vi "MicroStruct-XY.vi"() -> ()   [LabVIEW 2014]
doc: "Newport Motion Controler\nThis program make lines structure\n\nAndré Romero - 2020\nandretec@ifsc.usp.br"
uses:
  <vilib>/Platform/TimedLoop/XDataNode/timing_clust.ctl
  <vilib>/Platform/TimedLoop/XDataNode/nitl_modes.ctl
  <vilib>/Platform/TimedLoop/XDataNode/wakeup.ctl
  Basic-VIs/Global Motor Axis.vi
  <vilib>/Platform/TimedLoop/XDataNode/XDataNode.xnode
  <userlib>/Newport ESP301/Newport ESP301.lvlib
  <vilib>/Platform/TimedLoop/XDataNode/XDNodeRunTimeDep.lvlib
panel:
  out "Abort":bool
  out "current cycle":i32=1
  in  "Swap motor":bool=TRUE
  out "XY Graph":cluster{dbl[], dbl[]}(graph)={[0.0, 0.0, 0.002, 0.0105, 0.0215, 0.037, 0.0555, 0.075, 0.096, 0.116, 0.136, 0.156, 0.176, 0.1955, 0.216, 0.236, 0.256, 0.276, 0.2965, 0.3165, 0.336, 0.3565, 0.3755, 0.3965, 0.4165, 0.4365, 0.4565, 0.477, 0.4965, 0.5165, 0.5365, 0.557, 0.5765, 0.597, 0.617, 0.6365, 0.6565, 0.6765, 0.697, 0.717, 0.737, 0.757, 0.777, 0.797, 0.8165, 0.8375, 0.8575, 0.877, 0.897, 0.9175, 0.937, 0.9575, 0.977, 0.9975, 1.0005, 1.0005, 1.0, 0.997, 0.9885, 0.9775, 0.9615, 0.9435, 0.923, 0.903, 0.883, 0.863, 0.843, 0.823, 0.8035, 0.783, 0.763, 0.743, 0.723, 0.7035, 0.683, 0.6635, 0.643, 0.6235, 0.603, 0.583, 0.563, 0.543, 0.523, 0.5025, 0.483, 0.463, 0.443, 0.4225, 0.403, 0.3825, 0.363, 0.3425, 0.323, 0.303, 0.2825, 0.2625, 0.2425, 0.2225, 0.202, 0.183, 0.162, 0.1425, 0.1225, 0.1025, 0.082, 0.0625, 0.042, 0.0225, 0.002, -0.0005, -0.0005, 0.0, 0.0035, 0.013, 0.025, 0.0415, 0.06, 0.08, 0.1005, 0.1205, 0.1405, 0.1605, 0.18, 0.2005, 0.2205, 0.2405, 0.2605, 0.28, 0.3, 0.3205, 0.3405, 0.3605, 0.3805, 0.4005, 0.4205, 0.4405, 0.4605, 0.4805, 0.5005, 0.52, 0.541, 0.5605, 0.58, 0.6005, 0.6205, 0.6405, 0.6605, 0.6805, 0.7005, 0.7205, 0.7405, 0.7605, 0.7805, 0.8005, 0.8205, 0.8405, 0.8605, 0.8805, 0.9005, 0.92, 0.94, 0.96, 0.9805, 1.0005, 1.0005, 1.0005, 0.9995, 0.993, 0.984, 0.9705, 0.9535, 0.9335, 0.9135, 0.8935, 0.8735, 0.8535, 0.8335, 0.8135, 0.7935, 0.7735, 0.753, 0.7335, 0.713, 0.6935, 0.6735, 0.6535, 0.633, 0.6135], [0.0035, 0.0035, 0.0035, 0.0035, 0.0035, 0.0035, 0.0035, 0.0035, 0.0035, 0.0035, 0.0035, 0.0035, 0.0035, 0.0035, 0.0035, 0.0035, 0.0035, 0.0035, 0.0035, 0.0035, 0.0035, 0.0035, 0.0035, 0.0035, 0.0035, 0.0035, 0.0035, 0.0035, 0.0035, 0.0035, 0.0035, 0.0035, 0.0035, 0.0035, 0.0035, 0.0035, 0.0035, 0.0035, 0.0035, 0.0035, 0.0035, 0.0035, 0.0035, 0.0035, 0.0035, 0.0035, 0.0035, 0.0035, 0.0035, 0.0035, 0.0035, 0.0035, 0.0035, 0.0035, 0.0035, 0.004, 0.005, 0.0055, 0.0055, 0.0055, 0.0055, 0.006, 0.0055, 0.0055, 0.0055, 0.0055, 0.0055, 0.0055, 0.0055, 0.0055, 0.0055, 0.0055, 0.0055, 0.0055, 0.0055, 0.0055, 0.0055, 0.0055, 0.0055, 0.0055, 0.0055, 0.0055, 0.0055, 0.0055, 0.0055, 0.0055, 0.0055, 0.0055, 0.0055, 0.0055, 0.0055, 0.0055, 0.0055, 0.0055, 0.0055, 0.0055, 0.0055, 0.0055, 0.0055, 0.0055, 0.0055, 0.0055, 0.0055, 0.0055, 0.0055, 0.0055, 0.0055, 0.0055, 0.0055, 0.0055, 0.006, 0.0085, 0.0085, 0.0085, 0.0075, 0.0075, 0.0075, 0.007, 0.007, 0.0075, 0.0075, 0.0075, 0.0075, 0.0075, 0.0075, 0.0075, 0.0075, 0.0075, 0.0075, 0.0075, 0.0075, 0.0075, 0.0075, 0.0075, 0.0075, 0.0075, 0.0075, 0.0075, 0.0075, 0.0075, 0.0075, 0.0075, 0.0075, 0.0075, 0.0075, 0.0075, 0.0075, 0.0075, 0.0075, 0.0075, 0.0075, 0.0075, 0.0075, 0.0075, 0.0075, 0.0075, 0.0075, 0.0075, 0.0075, 0.0075, 0.0075, 0.0075, 0.0075, 0.0075, 0.0075, 0.0085, 0.01, 0.01, 0.01, 0.01, 0.01, 0.0095, 0.0095, 0.0095, 0.0095, 0.0095, 0.0095, 0.0095, 0.0095, 0.0095, 0.0095, 0.0095, 0.009, 0.009, 0.0095, 0.0095, 0.0095, 0.0095]}
  in  "N Cycles":i32=100 min=1
  in  "Acceleration (0 units/s²)":dbl=0.1 min=0.0 format="%#.4g"
  in  "Velocity (units/s)":dbl=0.1 min=0.0 format="%#.4g"
  in  "d (mm)":dbl=2.0
  in  "L (mm)":dbl=1.0
  out "X Position (mm)":dbl=0.6135 format="%.6g"
  out "Y Position (mm)":dbl=0.0095 format="%.6g"
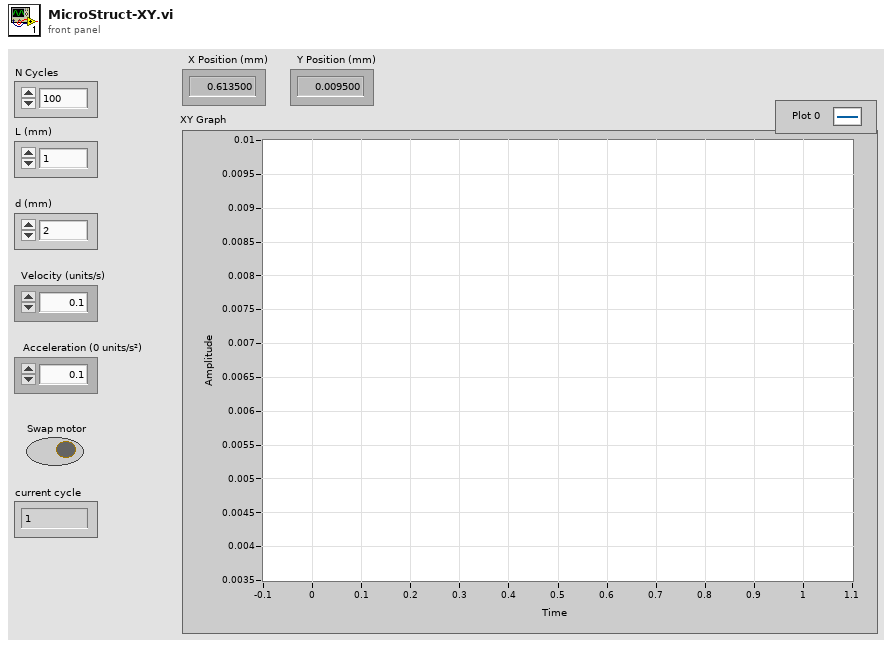
[diagram p1: front panel]
types:
  T1 = typedef "XDNodeRunTimeDep.lvlib/timing_clust.ctl" = cluster{"Expected End [f-1]":u64, "Actual End [f-1]":u64, "Finished Late? [f-1]":bool, "Expected End [i-1]":u64, "Actual End [i-1]":u64, "Finished Late? [i-1]":bool, "Expected Start [i]":u64, "Actual Start [i]":u64, "Expected Start [f]":u64, "Actual Start [f]":u64, "Source Name":string, "Structure Name":string, "Period":i64, "Deadline":i64, "Offset":i64, "Start":i64, "Priority":i32, "Timeout":i32, "Mode":T2, "Wakeup Reason":T3, "Error":errorcluster, "Source Type":string, "Secondary Source Type":string, "Global End Time":u64, "Global Start Time":u64, "Frame Duration":u64, "Iteration Duration":u64, "Assigned CPU":i32, "I/O Scan Engine Mode":u32}
  T2 = typedef "XDNodeRunTimeDep.lvlib/nitl_modes.ctl" = enum32{"No Change", "Process missed periods, maintain original phase", "Discard missed periods, maintain original phase", "Process missed periods, ignore original phase", "Discard missed periods, ignore original phase"}
  T3 = typedef "XDNodeRunTimeDep.lvlib/wakeup.ctl" = enum32{"Normal", "Aborted", "Asynchronous wakeup", "Timing source error", "Timed loop error", "Timeout"}
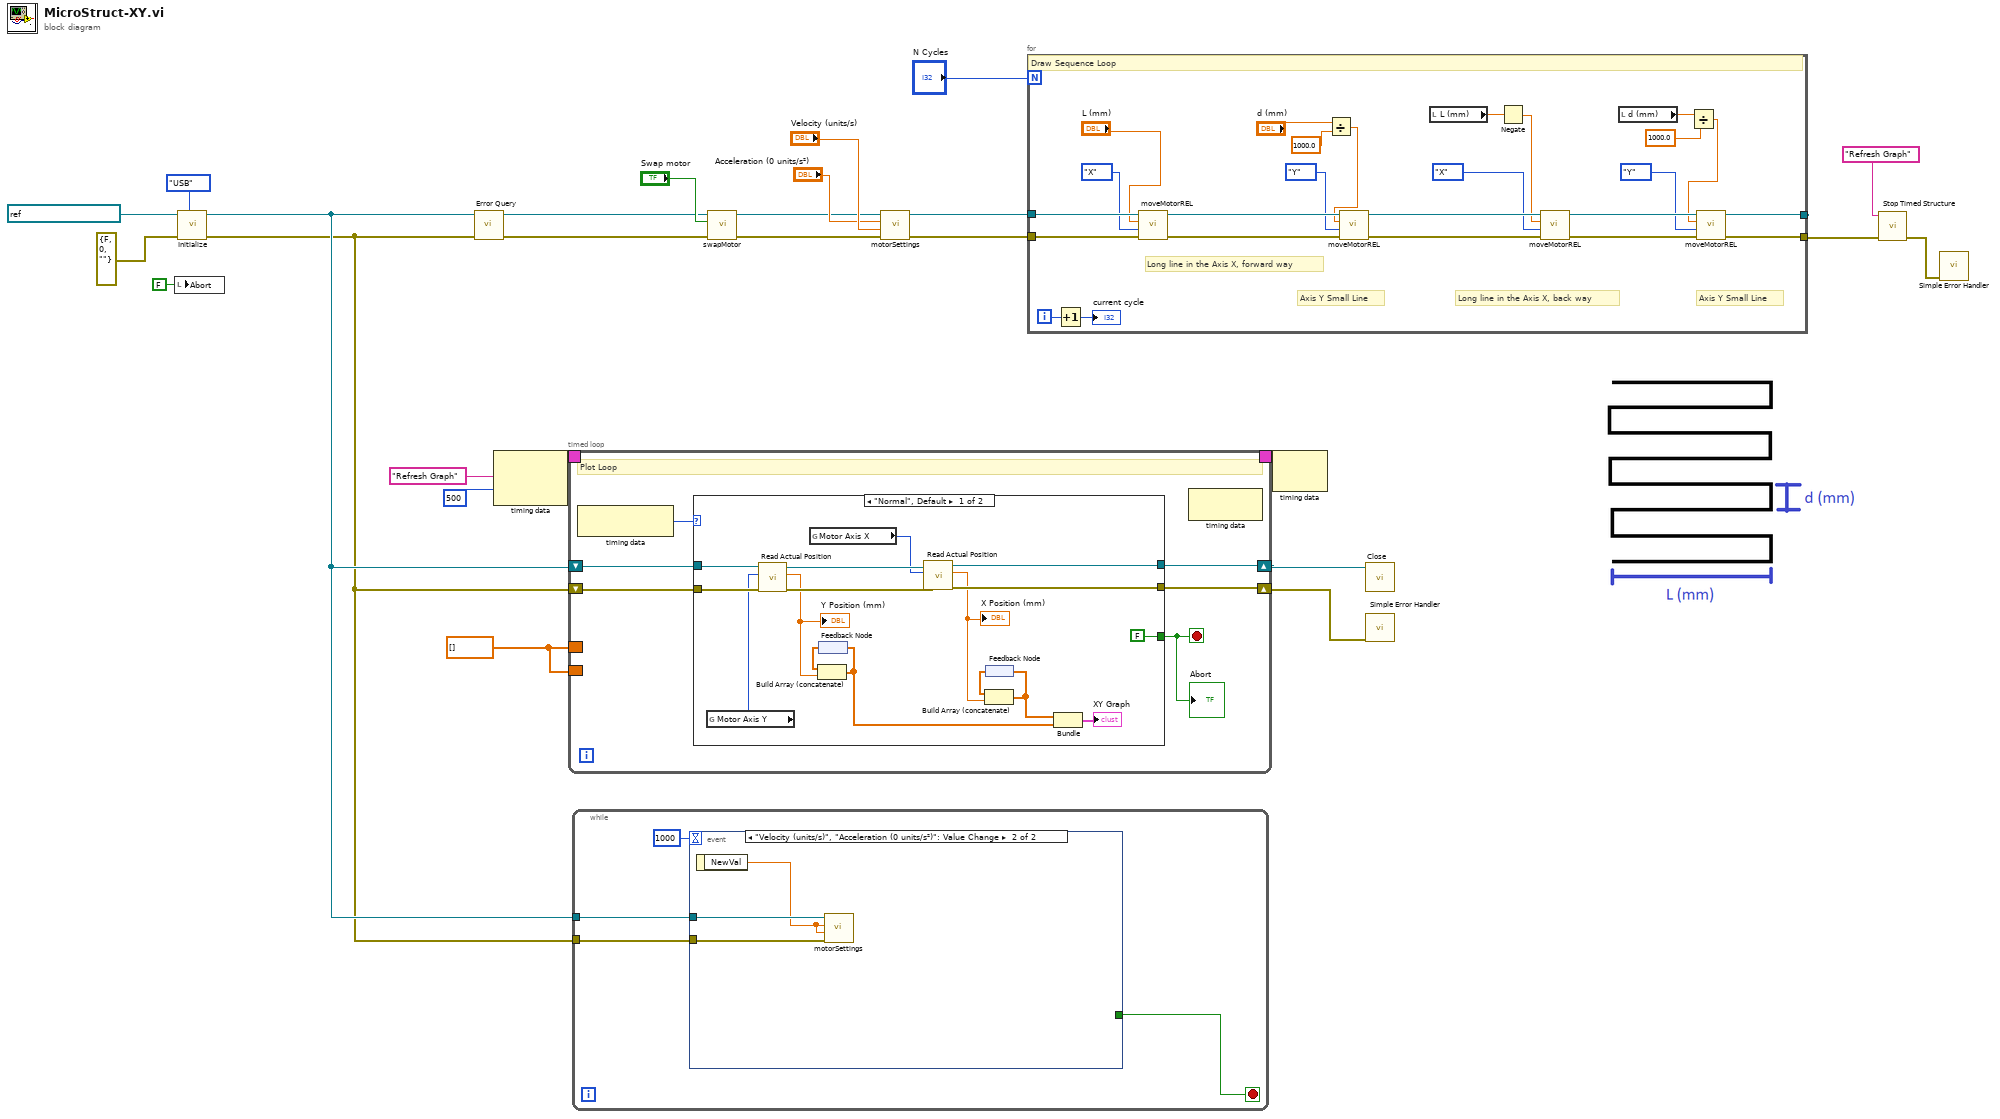
[diagram p0: block diagram]
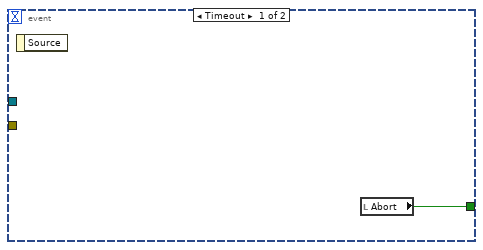
[diagram p2: hidden frame]
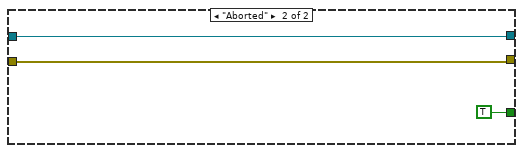
[diagram p3: hidden frame]
diagram:
  w14 = dbl[] []
  n1 = local write "Abort"(FALSE ("Abort")) -> ()
  n2 = call <userlib>:"Initialize.vi"("VISA resource name"=refnum<visa-resource-name> "ASRL3::INSTR" ("VISA resource name (duplicate)"), "error in (no error)"=errorcluster {"status"=FALSE, "code"=0, "source"=""}, "Serial Link (RS232)"=enum16{"RS232", "USB"}."USB") -> ("VISA resource name out"=w3:refnum<visa-resource-name>, "error out"=w2:errorcluster)  [unwired: 6 in]
  n3 = call <userlib>:"Error Query.vi"("error in (no error)"=w2, "VISA resource name"=w3) -> ("error out"=w9:errorcluster, "VISA resource name out"=w10:refnum<visa-resource-name>)  [unwired: 2 in, 2 out]
  n4 = node-c288("Refresh Graph" ("Structure Name"), i64 500 ("Period")) -> (w24:T1)
  n5 = timed-loop {
    timing: w24 -> [_]
    timing-out: [_] -> w23
    shift-right: [w30] -> w26
    shift-left: w3 -> [w32]
    shift-right: [w29] -> w25
    shift-left: w2 -> [w31]
    border: w14 -> [_]
    border: w14 -> [_]
    stop <- w27 stop-if-true
    # "Plot Loop"
    n6 = node-c288() -> (w28:T3)  [unwired: 1 in]
    n7 = case shown="\"Normal\", Default" w28 {
      tunnel: w32 -> [w48 w50]
      tunnel: w31 -> [w47 w49]
      tunnel: [w44 w50] -> w30
      tunnel: [w43 w49] -> w29
      tunnel: [FALSE TRUE] -> w27
      frame "Normal", Default {
        n8 = global read "Global Motor Axis.vi" "Motor Axis Y"() -> (w33:i32)
        n9 = call <userlib>:"Read Actual Position.vi"("error in (no error)"=w47, "Axis (1)"=w33, "VISA resource name"=w48) -> ("error out"=w45:errorcluster, "Position (units)"=w38:dbl, "VISA resource name out"=w46:refnum<visa-resource-name>)  [unwired: 2 in]
        "Y Position (mm)" <- w38
        n10 = global read "Global Motor Axis.vi" "Motor Axis X"() -> (w34:i32)
        n11 = feedback #1() -> (w41:dbl[])
        n12 = Build Array (concatenate)(w41, w38) -> (w36:dbl[])
        n13 = feedback-in #1(w36) -> ()
        n14 = call <userlib>:"Read Actual Position.vi"("error in (no error)"=w45, "Axis (1)"=w34, "VISA resource name"=w46) -> ("error out"=w43:errorcluster, "Position (units)"=w39:dbl, "VISA resource name out"=w44:refnum<visa-resource-name>)  [unwired: 2 in]
        "X Position (mm)" <- w39
        n15 = feedback #2() -> (w40:dbl[])
        n16 = Build Array (concatenate)(w40, w39) -> (w37:dbl[])
        n17 = feedback-in #2(w37) -> ()
        n18 = Bundle(w37, w36) -> (→"XY Graph":cluster{dbl[], dbl[]})  [unwired: 1 in]
      }
      frame "Aborted" {
      }
    }
    "Abort" <- w27
    n19 = node-c288() -> ()  [unwired: 1 in, 1 out]
  }
  n20 = while {
    tunnel: w3 -> [w58]
    tunnel: w2 -> [w57]
    stop <- w56 stop-if-true
    n21 = event shown="[1] \"Velocity (units/s)\", \"Acceleration (0 units/s²)\": Value Change" {
      selector: _ -> [_ _]
      dyn-events: _ -> [_ _]
      timeout: 1000 -> [_ _]
      tunnel: w58 -> [_ w61]
      tunnel: w57 -> [_ w62]
      tunnel: [w59 _] -> w56
      event Timeout {
        n22 = event-data() -> ()  [unwired: 1 in, 1 out]
        n23 = local read "Abort"() -> (w59:bool)
      }
      event "Velocity (units/s)", "Acceleration (0 units/s²)": Value Change {
        n24 = event-data() -> ("NewVal"=w60:dbl)  [unwired: 1 in]
        n25 = call "motorSettings.vi"("error in (no error)"=w62, "Velocity (units/s)"=w60, "Acceleration (0 units/s²)"=w60, "VISA Refnum in"=w61) -> ()  [unwired: 6 in, 2 out]
      }
    }
  }
  n26 = call "swapMotor.vi"("error in (no error)"=w9, "Swap motor"="Swap motor", "VISA Refnum in"=w10) -> ("error out"=w7:errorcluster, "VISA Refnum out"=w8:refnum<visa-resource-name>)  [unwired: 7 in]
  n27 = call "motorSettings.vi"("error in (no error)"=w7, "Velocity (units/s)"="Velocity (units/s)", "Acceleration (0 units/s²)"="Acceleration (0 units/s²)", "VISA Refnum in"=w8) -> ("error out"=w18:errorcluster, "VISA Refnum out"=w19:refnum<visa-resource-name>)  [unwired: 6 in]
  n28 = for {
    N: "N Cycles" -> [_]
    tunnel: w19 -> [w87]
    tunnel: w18 -> [w86]
    tunnel: [w75] -> _
    tunnel: [w74] -> w13
    i -> [w64]
    # "Axis Y Small Line"
    # "Long line in the Axis X, back way"
    # "Axis Y Small Line"
    # "Long line in the Axis X, forward way"
    # "Draw Sequence Loop"
    n29 = Increment(x=w64) -> (x+1=→"current cycle":i32)
    n30 = call "moveMotorREL.vi"("error in (no error)"=w86, "Axis"=enum16{"X", "Y"}."X", "L (mm)"="L (mm)", "VISA Refnum in"=w87) -> ("error out"=w83:errorcluster, "VISA Refnum out"=w84:refnum<visa-resource-name>)  [unwired: 6 in]
    n31 = Divide(x="d (mm)", y=1000.0 ("x")) -> (x/y=w68:dbl)
    n32 = call "moveMotorREL.vi"("error in (no error)"=w83, "Axis"=enum16{"X", "Y"}."Y", "L (mm)"=w68, "VISA Refnum in"=w84) -> ("error out"=w80:errorcluster, "VISA Refnum out"=w81:refnum<visa-resource-name>)  [unwired: 6 in]
    n33 = local read "L (mm)"() -> (w73:dbl)
    n34 = Negate(x=w73) -> (-x=w71:dbl)
    n35 = call "moveMotorREL.vi"("error in (no error)"=w80, "Axis"=enum16{"X", "Y"}."X", "L (mm)"=w71, "VISA Refnum in"=w81) -> ("error out"=w77:errorcluster, "VISA Refnum out"=w78:refnum<visa-resource-name>)  [unwired: 6 in]
    n36 = local read "d (mm)"() -> (w69:dbl)
    n37 = Divide(x=w69, y=1000.0) -> (x/y=w66:dbl)
    n38 = call "moveMotorREL.vi"("error in (no error)"=w77, "Axis"=enum16{"X", "Y"}."Y", "L (mm)"=w66, "VISA Refnum in"=w78) -> ("error out"=w74:errorcluster, "VISA Refnum out"=w75:refnum<visa-resource-name>)  [unwired: 6 in]
  }
  n39 = node-c288(w23) -> ()  [unwired: 1 out]
  n40 = call <userlib>:"Close.vi"("VISA resource name"=w26) -> ()  [unwired: 10 in, 1 out]
  n41 = call <vilib>:"Simple Error Handler.vi"("error in (no error)"=w25) -> ()  [unwired: 1 in, 8 out]
  n42 = call <vilib>:"Stop Timed Structure.vi"("error in (no error)"=w13, "name"="Refresh Graph" ("Structure Name")) -> ("error out"=w12:errorcluster)  [unwired: 9 in]
  n43 = call <vilib>:"Simple Error Handler.vi"("error in (no error)"=w12) -> ()  [unwired: 4 in, 5 out]
